vi "Litremeter top level v2.vi"() -> ()   [LabVIEW 2011]
panel:
  out "Sample DateTime":timestamp=timestamp(3418633364.71875 s since 1904-01-01)
  out "Time to fill (min)":dbl=-inf
  out "Fill rate":dbl(graph)
  out "Fill vol":dbl(graph)=13569.0
  in  "Tank capacity (L)":dbl=10000.0
  out "status":bool=TRUE
  out "Tank fill (%)":dbl(slide)=135.69 scale=0.0..100.0
  in  "Continuous measurement":bool=TRUE
  out "status":bool
  out "Litres":dbl=13569.0
  out "Pulses":u32=13569
  in  "Single-shot measurement":bool
  in  "Default Litres / pulse cal. factor":dbl=1.0
  in  "Litres / pulse":dbl=1.0
  in  "Specify Litres / pulse cal. factor":bool
  in  "offset (L)":dbl
  in  "Specify fill offset":bool
  in  "Refresh rate (Hz)":dbl=10.0
  in  "stop":bool
  out "status":bool=TRUE
  in  "Counter":tag="Dev2/ctr0"
  in  "Device":tag="Dev2"
  in  "Enable counter":bool=TRUE
  # "Paul Nathan, 02/03/2012"
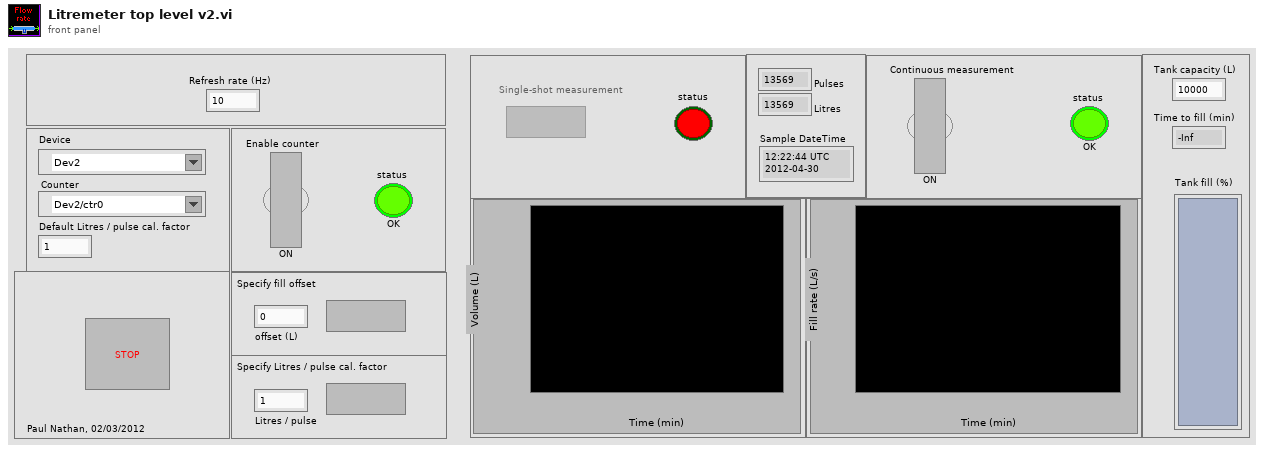
[diagram p1: front panel]
types:
  T1 = enum8{"Enabled", "Disabled", "Disabled and Grayed Out"}
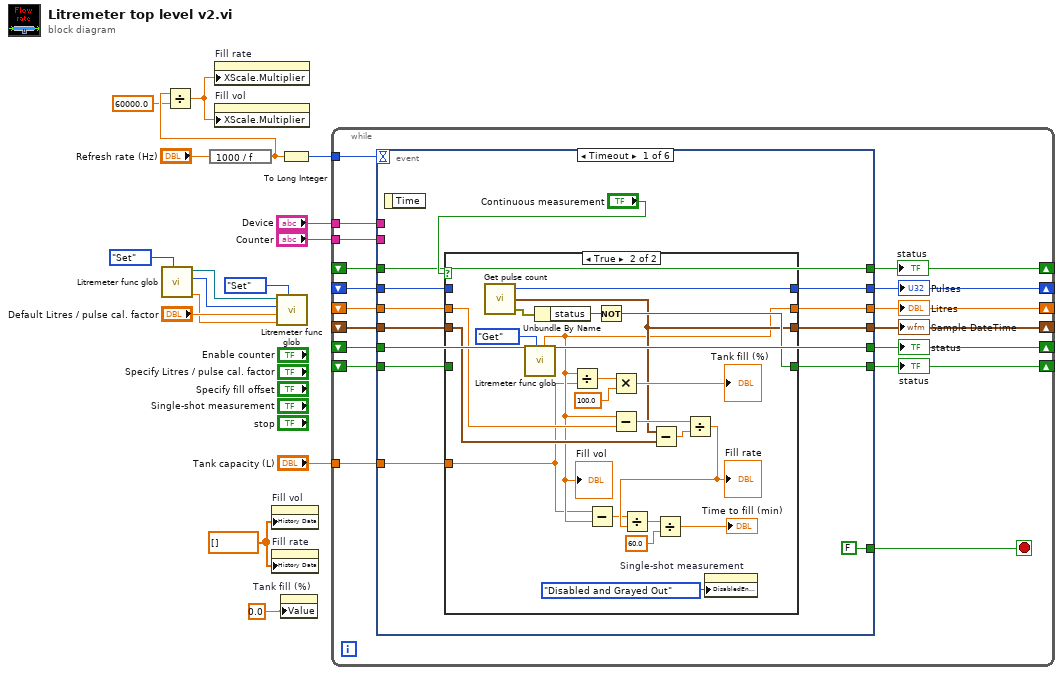
[diagram p0: block diagram]
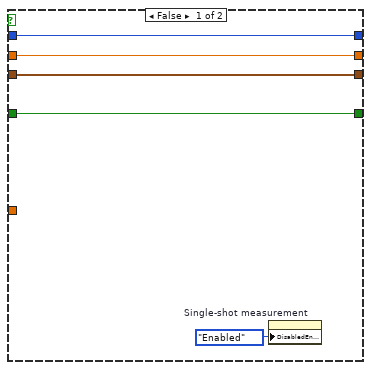
[diagram p2: hidden frame]
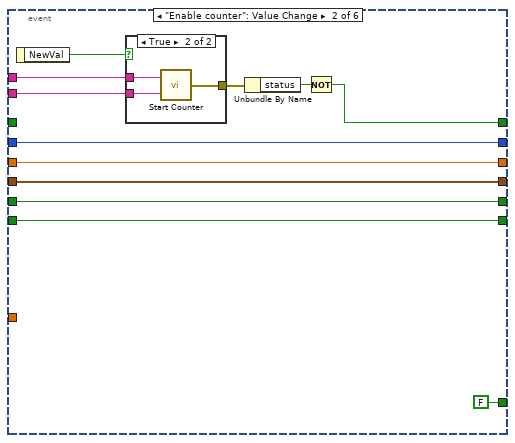
[diagram p3: hidden frame]
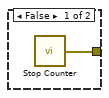
[diagram p4: hidden frame]
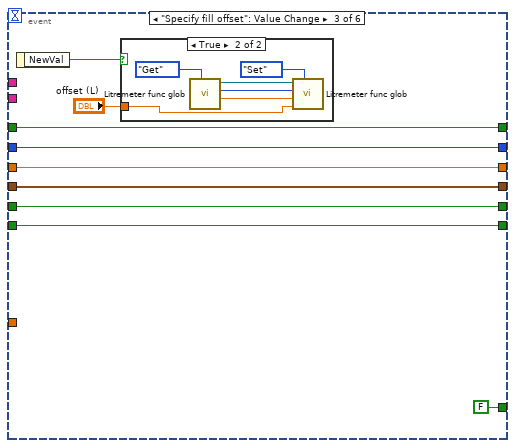
[diagram p5: hidden frame]
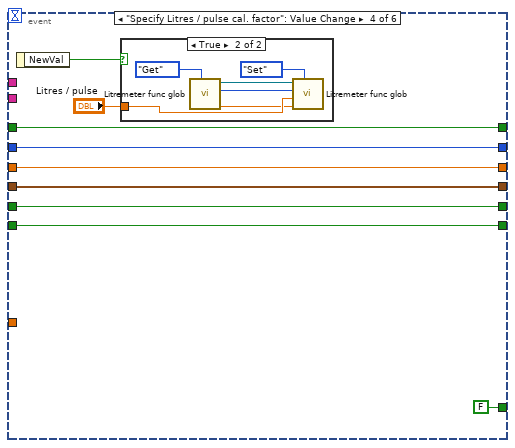
[diagram p7: hidden frame]
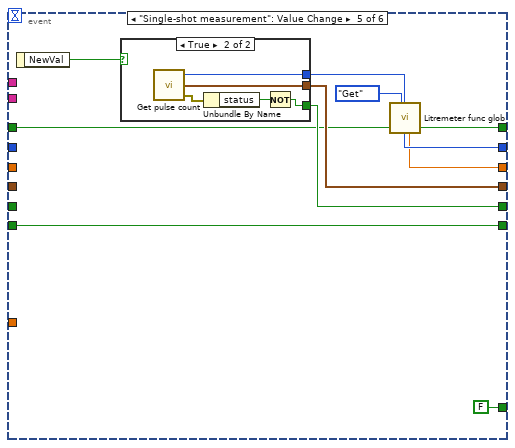
[diagram p9: hidden frame]
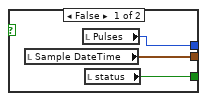
[diagram p10: hidden frame]
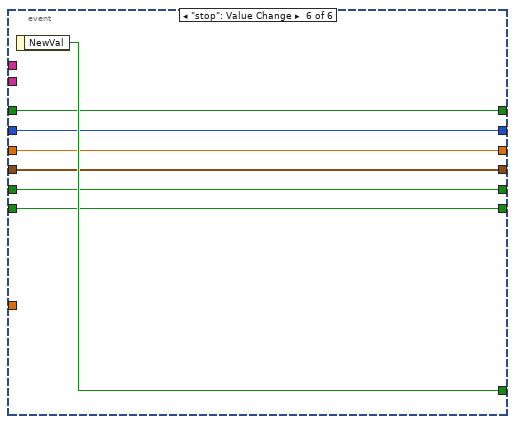
[diagram p11: hidden frame]
diagram:
  w5 = dbl[] [] ("History Data")
  n1 = call "Litremeter func glob.vi"("Action"=enum16{"Get", "Set"}."Set") -> ("Offset Litres out"=w10:dbl, "Pulse count out"=w9:u32, "Counter task out"=w8:refnum<k21>)  [unwired: 4 in, 2 out]
  n2 = expression code="1000 / f"("Refresh rate (Hz)") -> (w2:dbl)
  n3 = Divide(x=w2, y=60000.0) -> (x/y=w3:dbl)
  n4 = property on="Fill rate" class="WFChart (strict)"("XScale.Multiplier"=w3) -> ()  [unwired: 2 in, 2 out]
  n5 = property on="Fill vol" class="WFChart (strict)"("XScale.Multiplier"=w3) -> ()  [unwired: 2 in, 2 out]
  n6 = property on="Fill vol" class="WFChart (strict)"("History Data"=w5) -> ()  [unwired: 2 in, 2 out]
  n7 = property on="Fill rate" class="WFChart (strict)"("History Data"=w5) -> ()  [unwired: 2 in, 2 out]
  n8 = call "Litremeter func glob.vi"("Action"=enum16{"Get", "Set"}."Set", "Offset Litres in"=w10, "Litres / pulse in"="Default Litres / pulse cal. factor", "Pulse count in"=w9, "Counter task in"=w8) -> ()  [unwired: 5 out]
  n9 = To Long Integer(number=w2) -> (32bit integer=w7:i32)
  n10 = property on="Tank fill (%)" class="Slide (strict)"("Value"=0.0 ("Tank fill (%)")) -> ()  [unwired: 2 in, 2 out]
  n11 = while {
    tunnel: "Device" -> [w33]
    tunnel: "Counter" -> [w32]
    tunnel: w7 -> [w31]
    tunnel: "Tank capacity (L)" -> [w27]
    shift-right: [w29] -> _
    shift-left: _ -> [w28]
    shift-right: [w23] -> _
    shift-left: _ -> [w17]
    shift-right: [w22] -> _
    shift-left: _ -> [w18]
    shift-right: [w21] -> _
    shift-left: _ -> [w26]
    shift-right: [w25] -> _
    shift-left: _ -> [w24]
    shift-right: [w20] -> _
    shift-left: _ -> [w19]
    stop <- w30 stop-if-true
    n12 = event shown="[0] Timeout" {
      selector: _ -> [_ _ _ _ _ _]
      dyn-events: _ -> [_ _ _ _ _ _]
      timeout: w31 -> [_ _ _ _ _ _]
      tunnel: w33 -> [_ w84 _ _ _ _]
      tunnel: w32 -> [_ w83 _ _ _ _]
      tunnel: [w34 w79 w94 w109 w119 w141] -> w23
      tunnel: [w40 w73 w93 w108 w125 w140] -> w22
      tunnel: [w38 w77 w92 w107 w124 w139] -> w21
      tunnel: [w43 w76 w91 w106 w123 w138] -> w29
      tunnel: [w35 w75 w90 w105 w122 w137] -> w25
      tunnel: [FALSE ("NewVal") FALSE ("NewVal") FALSE ("NewVal") FALSE ("NewVal") FALSE ("NewVal") w142] -> w30
      tunnel: w28 -> [w44 w76 w91 w106 _ w138]
      tunnel: w27 -> [w42 _ _ _ _ _]
      tunnel: [w41 w74 w89 w104 w120 w136] -> w20
      tunnel: w26 -> [w39 w77 w92 w107 _ w139]
      tunnel: w24 -> [w35 w75 w90 w105 _ w137]
      tunnel: w19 -> [w37 w74 w89 w104 w120 w136]
      tunnel: w18 -> [w36 w73 w93 w108 _ w140]
      tunnel: w17 -> [w34 _ w94 w109 w119 w141]
      event Timeout {
        n13 = event-data() -> ()  [unwired: 1 in, 1 out]
        n14 = case shown="True" "Continuous measurement" {
          tunnel: [w48 w72] -> w40
          tunnel: [w49 w60] -> w43
          tunnel: [w51 w69] -> w41
          tunnel: [w50 w54] -> w38
          tunnel: w42 -> [_ w53]
          tunnel: w39 -> [w50 w64]
          tunnel: w44 -> [w49 w62]
          tunnel: w37 -> [w51 _]
          tunnel: w36 -> [w48 _]
          frame False {
            n15 = property on="Single-shot measurement" class="Bool (strict)"("DisabledEnum"=T1."Enabled" ("Disabled")) -> ()  [unwired: 2 in, 2 out]
          }
          frame True {
            n16 = call "Get pulse count.vi"() -> ("Error"=w70:errorcluster, "Sample DateTime"=w60:timestamp, "Pulse count"=w72:u32)
            n17 = call "Litremeter func glob.vi"("Action"=enum16{"Get", "Set"}."Get") -> ("Total Litres (calc)"=w54:dbl)  [unwired: 4 in, 4 out]
            "Fill vol" <- w54
            n18 = Unbundle By Name(w70) -> ("status"=w71:bool)
            n19 = Divide(x=w54, y=w53) -> (x/y=w66:dbl)
            n20 = Subtract(x=w53, y=w54) -> (x-y=w52:dbl)
            n21 = Not(x=w71) -> (.not. x?=w69:bool)
            n22 = Multiply(x=w66, y=100.0 ("x")) -> (x*y=→"Tank fill (%)":dbl)
            n23 = Subtract(x=w54, y=w64) -> (x-y=w63:dbl)
            n24 = Subtract(x=w60, y=w62) -> (x-y=w61:dbl)
            n25 = Divide(x=w63, y=w61) -> (x/y=w59:dbl)
            "Fill rate" <- w59
            n26 = Divide(x=w52, y=w59) -> (x/y=w58:dbl)
            n27 = Divide(x=w58, y=60.0) -> (x/y=→"Time to fill (min)":dbl)
            n28 = property on="Single-shot measurement" class="Bool (strict)"("DisabledEnum"=T1."Disabled and Grayed Out" ("Disabled")) -> ()  [unwired: 2 in, 2 out]
          }
        }
      }
      event "Enable counter": Value Change {
        n29 = event-data() -> ("NewVal"=w82:bool)  [unwired: 1 in]
        n30 = case shown="True" w82 {
          tunnel: w84 -> [_ w88]
          tunnel: w83 -> [_ w87]
          tunnel: [w85 w86] -> w80
          frame False {
            n31 = call "Stop Counter.vi"() -> ("Error"=w85:errorcluster)
          }
          frame True {
            n32 = call "Start Counter.vi"("Counter"=w87, "Device"=w88) -> ("Error"=w86:errorcluster)
          }
        }
        n33 = Unbundle By Name(w80) -> ("status"=w81:bool)
        n34 = Not(x=w81) -> (.not. x?=w79:bool)
      }
      event "Specify fill offset": Value Change {
        n35 = event-data() -> ("NewVal"=w97:bool)  [unwired: 1 in]
        n36 = case shown="True" w97 {
          tunnel: "offset (L)" -> [_ w99]
          frame False {
          }
          frame True {
            n37 = call "Litremeter func glob.vi"("Action"=enum16{"Get", "Set"}."Get") -> ("Litres / pulse out"=w100:dbl, "Pulse count out"=w98:u32, "Counter task out"=w101:refnum<k21>)  [unwired: 4 in, 2 out]
            n38 = call "Litremeter func glob.vi"("Action"=enum16{"Get", "Set"}."Set", "Offset Litres in"=w99, "Litres / pulse in"=w100, "Pulse count in"=w98, "Counter task in"=w101) -> ()  [unwired: 5 out]
          }
        }
      }
      event "Specify Litres / pulse cal. factor": Value Change {
        n39 = event-data() -> ("NewVal"=w111:bool)  [unwired: 1 in]
        n40 = case shown="True" w111 {
          tunnel: "Litres / pulse" -> [_ w116]
          frame False {
          }
          frame True {
            n41 = call "Litremeter func glob.vi"("Action"=enum16{"Get", "Set"}."Get") -> ("Offset Litres out"=w115:dbl, "Pulse count out"=w114:u32, "Counter task out"=w113:refnum<k21>)  [unwired: 4 in, 2 out]
            n42 = call "Litremeter func glob.vi"("Action"=enum16{"Get", "Set"}."Set", "Offset Litres in"=w115, "Litres / pulse in"=w116, "Pulse count in"=w114, "Counter task in"=w113) -> ()  [unwired: 5 out]
          }
        }
      }
      event "Single-shot measurement": Value Change {
        n43 = event-data() -> ("NewVal"=w126:bool)  [unwired: 1 in]
        n44 = case shown="True" w126 {
          tunnel: [w130 w135] -> w125
          tunnel: [w129 w134] -> w123
          tunnel: [w128 w131] -> w122
          frame False {
            n45 = local read "Sample DateTime"() -> (w129:timestamp)
            n46 = local read "Pulses"() -> (w130:u32)
            n47 = local read "status"() -> (w128:bool)
          }
          frame True {
            n48 = call "Get pulse count.vi"() -> ("Error"=w132:errorcluster, "Sample DateTime"=w134:timestamp, "Pulse count"=w135:u32)
            n49 = Unbundle By Name(w132) -> ("status"=w133:bool)
            n50 = Not(x=w133) -> (.not. x?=w131:bool)
          }
        }
        n51 = call "Litremeter func glob.vi"("Action"=enum16{"Get", "Set"}."Get") -> ("Total Litres (calc)"=w124:dbl)  [unwired: 4 in, 4 out]
      }
      event "stop": Value Change {
        n52 = event-data() -> ("NewVal"=w142:bool)  [unwired: 1 in]
      }
    }
    "status" <- w23
    "Pulses" <- w22
    "Litres" <- w21
    "status" <- w25
    "status" <- w20
    "Sample DateTime" <- w29
  }
